vi "SUB_GeCurrenttTime_String.vi"() -> (1 "concatenated string":string)   [LabVIEW 2011]
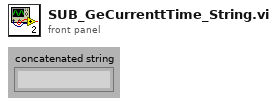
[diagram p1: front panel]
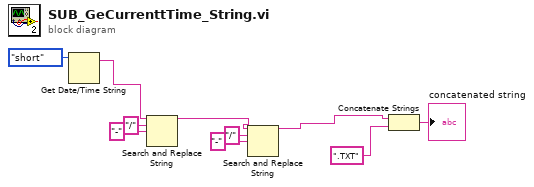
[diagram p0: block diagram]
diagram:
  n1 = Get Date/Time String(date format (0)=enum16{"short", "long", "abbreviated"}."short") -> (date string=w9:string)  [unwired: 2 in, 1 out]
  n2 = Search and Replace String(input string=w9, search string="/", replace string="-" ("replace string (\"\")")) -> (result string=w4:string)  [unwired: 5 in, 3 out]
  n3 = Search and Replace String(input string=w4, search string="/", replace string="-" ("replace string (\"\")")) -> (result string=w3:string)  [unwired: 5 in, 3 out]
  n4 = Concatenate Strings(w3, ".TXT") -> (→"concatenated string":string)
